vi "HRVcalc.vi"(9 "Time":dbl[](array[numeric]), 10 "Locations":dbl[](array[numeric]), 11 "2D":dbl[][](array[numeric])) -> (1 "XY Graph":cluster{dbl[], dbl[]}(graph), 2 "deltaPeakTimes":dbl[](array[numeric]), 3 "peakTimes":dbl[](array[numeric]))   [LabVIEW 2025]
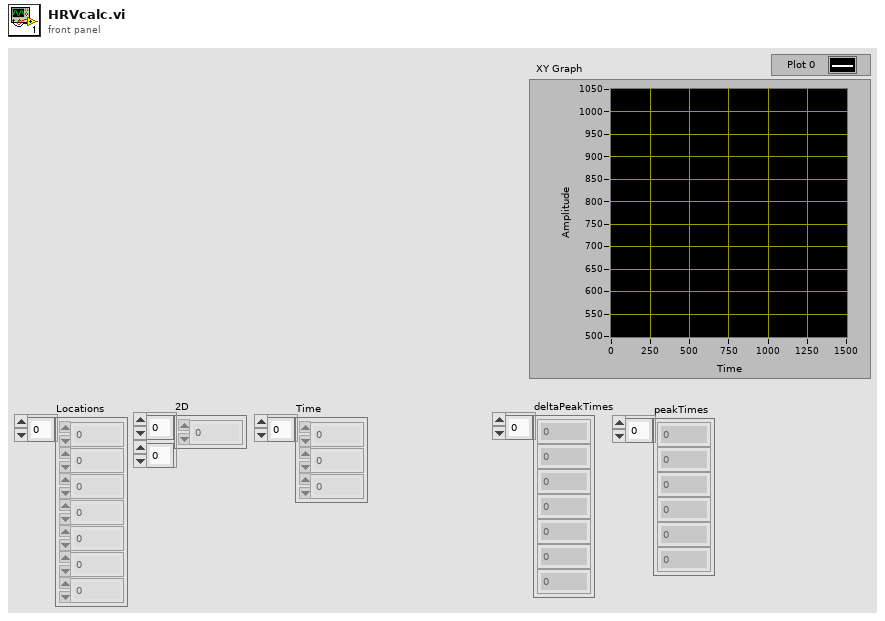
[diagram p1: front panel]
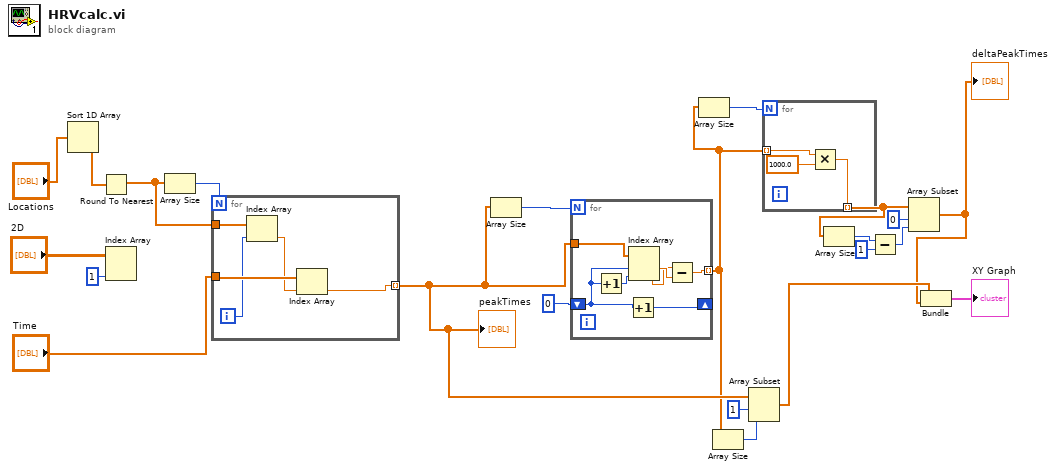
[diagram p0: block diagram]
diagram:
  n1 = Sort 1D Array(array="Locations") -> (sorted array=w8:dbl[])
  n2 = Round To Nearest(number=w8) -> (nearest integer value=w19:dbl[])
  n3 = Index Array(array="2D", index (col)=1 ("disabled index (col)")) -> ()  [unwired: 1 in, 1 out]
  n4 = Array Size(array=w19) -> (size(s)=w20:i32)
  n5 = for {
    N: w20 -> [_]
    tunnel: "Time" -> [w27]
    tunnel: w19 -> [w26]
    tunnel: [w23] -> w16 mode=indexing
    i -> [w25]
    n6 = Index Array(array=w26, index=w25) -> (element=w24:dbl)
    n7 = Index Array(array=w27, index=w24) -> (element=w23:dbl)
  }
  "peakTimes" <- w16
  n8 = Array Size(array=w16) -> (size(s)=w17:i32)
  n9 = for {
    N: w17 -> [_]
    tunnel: w16 -> [w34]
    tunnel: [w32] -> w7 mode=indexing
    shift-right: [w28] -> _
    shift-left: 0 -> [w29]
    n10 = Increment(x=w29) -> (x+1=w33:i32)
    n11 = Increment(x=w29) -> (x+1=w28:i32)
    n12 = Index Array(array=w34, index #1=w29, index #2=w33) -> (element #1=w31:dbl, element #2=w30:dbl)
    n13 = Subtract(x=w30, y=w31) -> (x-y=w32:dbl)
  }
  n14 = Array Size(array=w7) -> (size(s)=w10:i32)
  n15 = Array Size(array=w7) -> (size(s)=w14:i32)
  n16 = Array Subset(array=w16, index=1, length=w14) -> (w11:dbl[])
  n17 = for {
    N: w10 -> [_]
    tunnel: w7 -> [w37] mode=indexing
    tunnel: [w35] -> w5 mode=indexing
    n18 = Multiply(x=w37, y=1000.0) -> (x*y=w35:dbl)
  }
  n19 = Array Size(array=w5) -> (size(s)=w4:i32)
  n20 = Subtract(x=w4, y=1) -> (x-y=w2:i32)
  n21 = Array Subset(array=w5, index=0, length=w2) -> (w1:dbl[])
  "deltaPeakTimes" <- w1
  n22 = Bundle(w11, w1) -> (→"XY Graph":cluster{dbl[], dbl[]})  [unwired: 1 in]
